vi "Get Reserved Names.vi"() -> (2 "reserved names":string[](array[string])=["InstrumentStudioPluginSDK"])   [LabVIEW 2021, in "G Plugin Editor.lvlib"]
uses:
  G Plugin Editor.lvlib
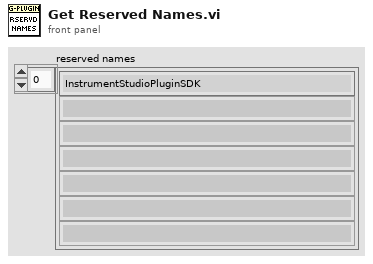
[diagram p1: front panel]
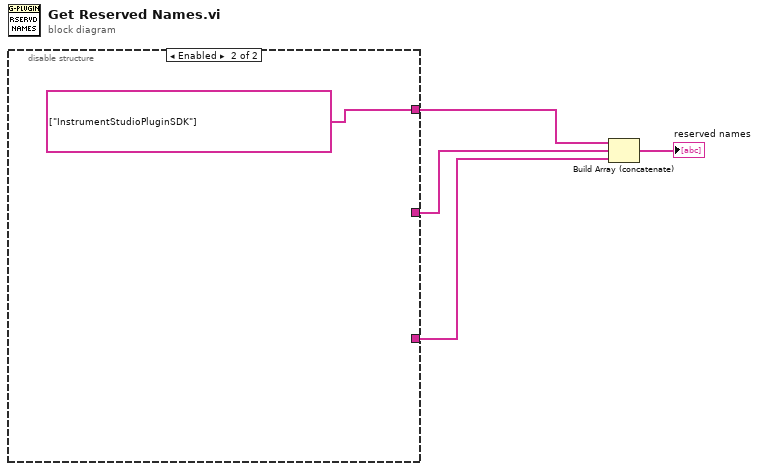
[diagram p0: block diagram]
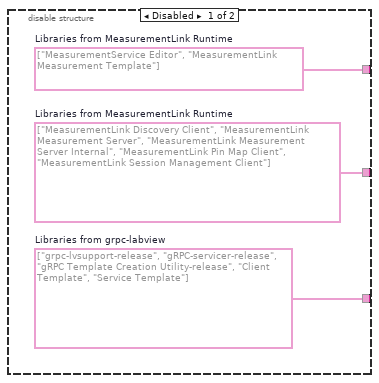
[diagram p2: hidden frame]
diagram:
  n1 = disable-structure shown="Enabled" {
    disable-tunnel: [w7 _] -> w4
    disable-tunnel: [w6 _] -> w3
    disable-tunnel: [w5 string[] ["InstrumentStudioPluginSDK"] ("Libraries from MeasurementLink Runtime")] -> w2
    frame Disabled {
      w5 = string[] ["MeasurementService Editor", "MeasurementLink Measurement Template"]  # Libraries from MeasurementLink Runtime
      w7 = string[] ["grpc-lvsupport-release", "gRPC-servicer-release", "gRPC Template Creation Utility-release", "Client Template", "Service Template"]  # Libraries from grpc-labview
      w6 = string[] ["MeasurementLink Discovery Client", "MeasurementLink Measurement Server", "MeasurementLink Measurement Server Internal", "MeasurementLink Pin Map Client", "MeasurementLink Session Management Client"]  # Libraries from MeasurementLink Runtime
    }
    frame Enabled {
    }
  }
  n2 = Build Array (concatenate)(w2, w3, w4) -> (→"reserved names":string[])
